vi "UdsLogEvent.vi"(0 "UdsHandleIn":T1, 2 "LogSuspend":bool, 5 "EventMsg":string, 11 "error in":errorcluster) -> (4 "UdsHandleOut":T1, 15 "error out":errorcluster)   [LabVIEW 2011, in "Konvolucio MUDS150628.lvlib"]
uses:
  <instrlib>/Konvolucio MUDS150628/Konvolucio MUDS150628.lvlib
  <instrlib>/Konvolucio MUDS150628/Types/UdsHandleType.ctl
  <instrlib>/Konvolucio MCAN120803/Types/MCanHandleType.ctl
  C:/Program Files/National Instruments/LabVIEW 2011/instr.lib/Konvolucio MCAN120803/Private/Konvolucio.MCAN120803.dll
  Konvolucio MCAN120803/Private/Konvolucio.MCAN120803.dll
  <instrlib>/Konvolucio MCAN120803/Konvolucio MCAN120803.lvlib
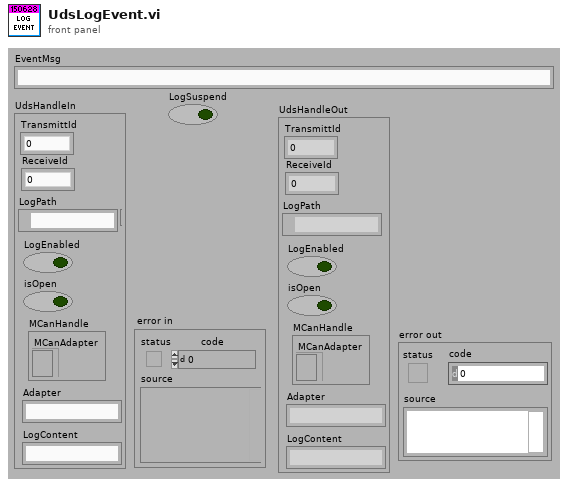
[diagram p1: front panel]
types:
  T1 = typedef "Konvolucio MUDS150628.lvlib/UdsHandleType.ctl" = cluster{"LogPath":path, "LogEnabled":bool, "isOpen":bool, "LogContent":string, "Adapter":string, "MCanHandle":T2, "TransmittId":u32, "ReceiveId":u32}
  T2 = typedef "Konvolucio MCAN120803.lvlib/MCanHandleType.ctl" = cluster{"MCanAdapter":refnum<k24>}
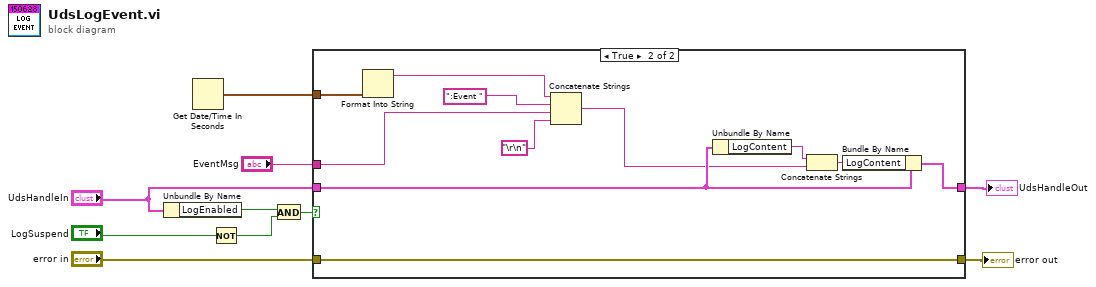
[diagram p0: block diagram]
diagram:
  n1 = Unbundle By Name("UdsHandleIn") -> ("LogEnabled"=w6:bool)
  n2 = Get Date/Time In Seconds() -> (seconds since 1Jan1904=w2:timestamp)
  n3 = Not(x="LogSuspend") -> (.not. x?=w4:bool)
  n4 = And(x=w6, y=w4) -> (x .and. y?=w3:bool)
  n5 = case shown="True" w3 {
    tunnel: "error in" -> [w12 w15]
    tunnel: [w12 w15] -> w9
    tunnel: [w11 w23] -> w7
    tunnel: "UdsHandleIn" -> [w11 w22]
    tunnel: w2 -> [_ w19]
    tunnel: "EventMsg" -> [_ w13]
    frame False {
    }
    frame True {
      n6 = Format Into String(w19) -> (resulting string=w17:string)  [unwired: 3 in, 1 out]
      n7 = Concatenate Strings(w17, ":Event " ("string"), w13, "\r\n") -> (w16:string)
      n8 = Unbundle By Name(w22) -> ("LogContent"=w20:string)
      n9 = Concatenate Strings(w20, w16) -> (w21:string)
      n10 = Bundle By Name(cluster=w22, "LogContent"=w21) -> (w23:T1)
    }
  }
  "error out" <- w9
  "UdsHandleOut" <- w7
